vi "ex9_data types.vi"() -> ()   [LabVIEW 2018]
panel:
  in  "String":string
  out "String 2":string
  in  "Cluster":T1
  out "Array 2":dbl[](array[numeric])
  in  "stop":bool
  out "Boolean 2":bool
  out "size(s)":i32
  out "Numeric 3":dbl
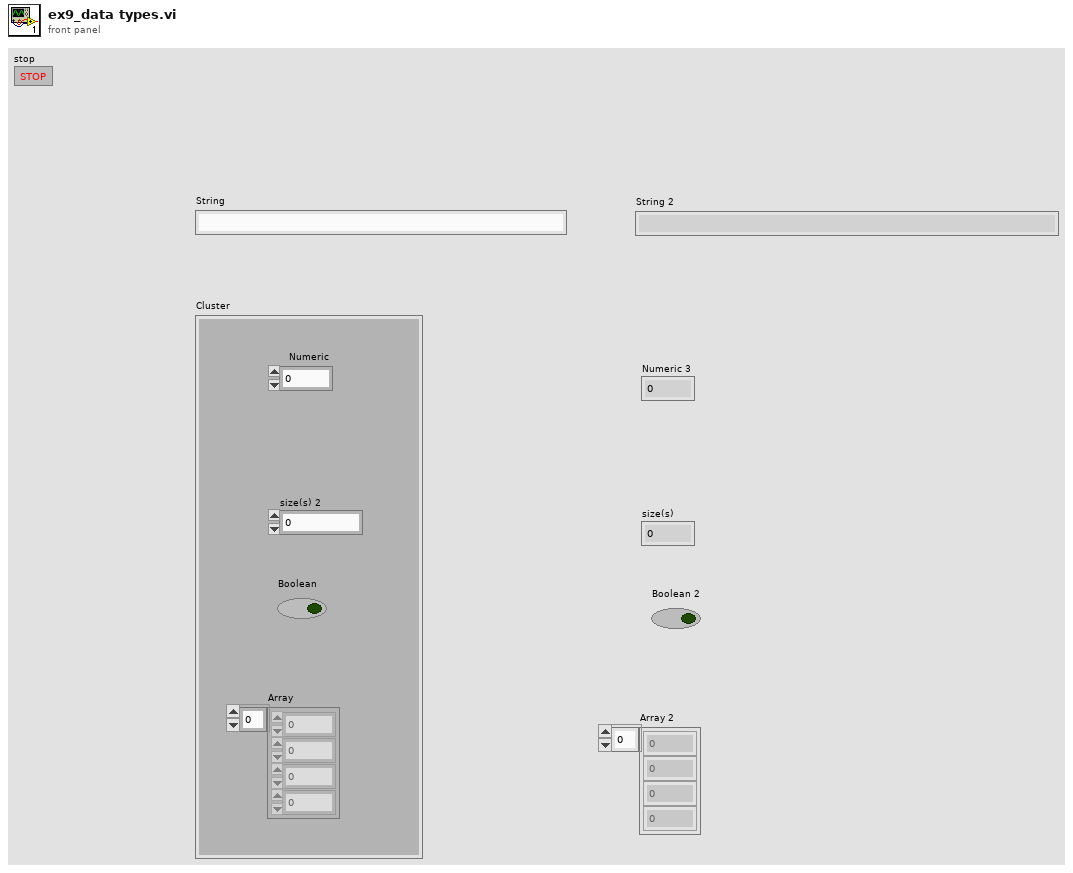
[diagram p1: front panel]
types:
  T1 = cluster{"Numeric":dbl, "size(s) 2":i32, "Boolean":bool, "Array":dbl[]}
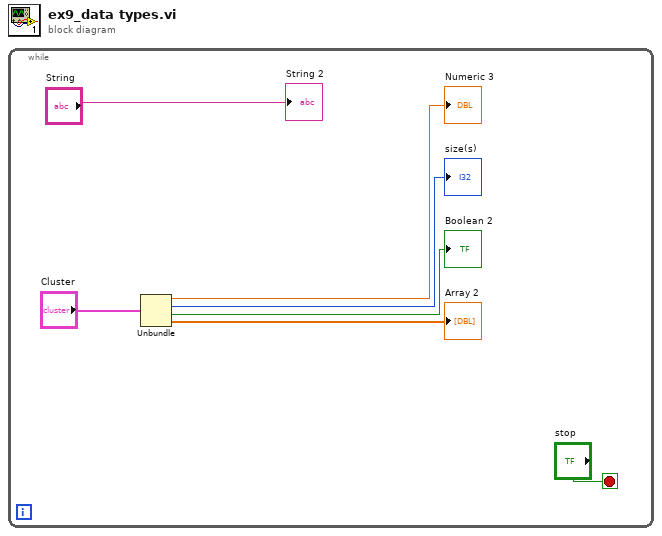
[diagram p0: block diagram]
diagram:
  n1 = while {
    stop <- "stop" stop-if-true
    n2 = Unbundle("Cluster") -> ("Numeric"=→"Numeric 3":dbl, "size(s) 2"=→"size(s)":i32, "Boolean"=→"Boolean 2":bool, "Array"=→"Array 2":dbl[])
    "String 2" <- "String"
  }
